vi "Sort Points.vi"(9 "Point 3":T1, 10 "Point 2":T1, 11 "Point 1":T1) -> (1 "Point 3":T1, 2 "Point 2":T1, 3 "Point 1":T1)   [LabVIEW 2020, in "Raster.lvlib"]
uses:
  Raster.lvlib
  Point 2D.ctl
  <userlib>/_OpenG.lib/array/array.llb/Sort 1D Array (I32)__ogtk.vi
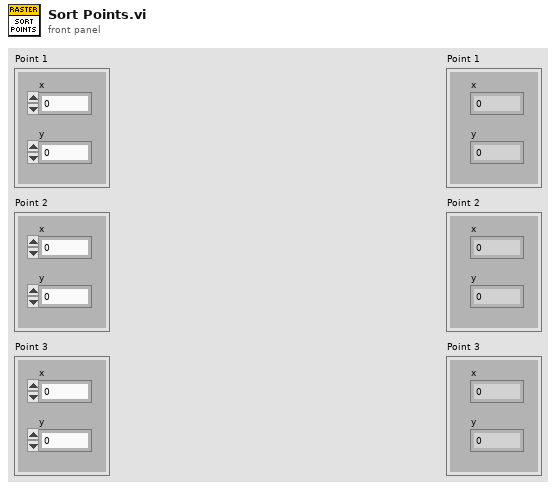
[diagram p1: front panel]
types:
  T1 = typedef "Raster.lvlib/Point 2D.ctl" = cluster{"x":i32, "y":i32}
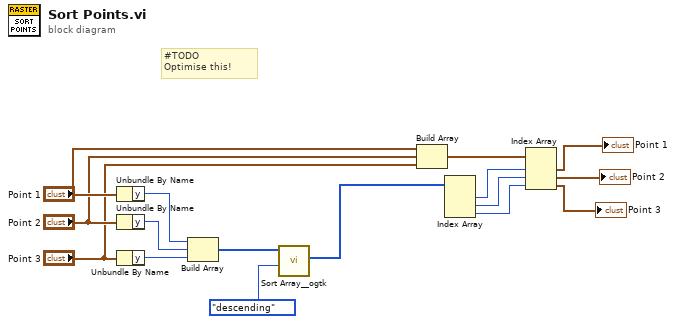
[diagram p0: block diagram]
diagram:
  # "#TODO\nOptimise this!"
  n1 = Unbundle By Name("Point 1") -> ("y"=w16:i32)
  n2 = Unbundle By Name("Point 2") -> ("y"=w15:i32)
  n3 = Unbundle By Name("Point 3") -> ("y"=w14:i32)
  n4 = Build Array(w16, w15, w14) -> (w13:i32[])
  n5 = call-poly <userlib>:"Sort Array__ogtk.vi"("Order"=enum16{"ascending", "descending"}."descending", "Array in"=w13) -> ("Sorted Pointers"=w5:i32[])  [unwired: 8 in, 1 out]
  n6 = Build Array("Point 1", "Point 2", "Point 3") -> (w9:T1[])
  n7 = Index Array(array=w5) -> (element #1=w4:i32, element #2=w3:i32, element #3=w2:i32)  [unwired: 3 in]
  n8 = Index Array(array=w9, index #1=w4, index #2=w3, index #3=w2) -> (element #1=→"Point 1":T1, element #2=→"Point 2":T1, element #3=→"Point 3":T1)
